vi "SequenceIndexGet.vi"(8 "error in (no error)":errorcluster, 10 "SequenceIndexName":string, 11 "VariableManager in":refnum<class "VariableManager.lvclass">) -> (0 "error out":errorcluster, 2 "SequenceIndex":refnum<class "SequenceIndex.lvclass">, 3 "VariableManager out":refnum<class "VariableManager.lvclass">)   [LabVIEW 2013, in "VariableManager.lvclass"]
doc: "Return sequence index definition of SequenceIndexName\n\nAn error is thrown if a SequenceIndexName does not exist."
uses:
  VariableManager.lvclass
  SequenceIndex/SequenceIndex.lvclass
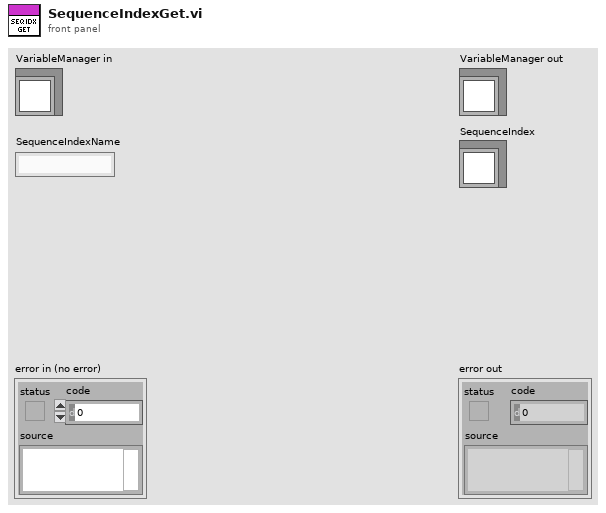
[diagram p1: front panel]
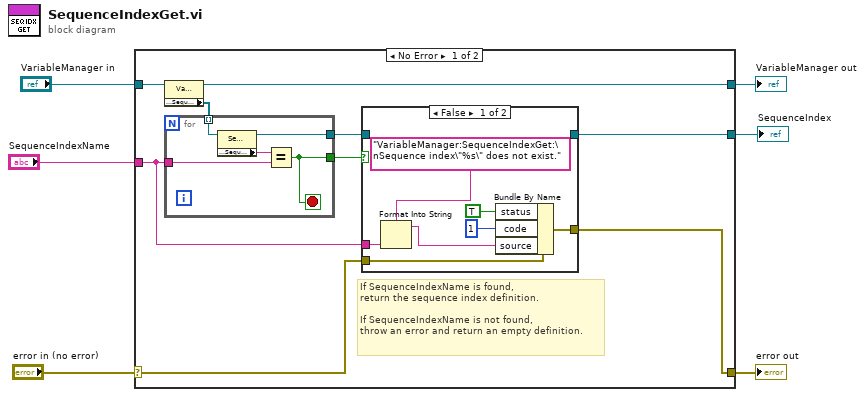
[diagram p0: block diagram]
diagram:
  n1 = case shown="No Error" "error in (no error)" {
    selector: "error in (no error)" -> [w9 w31]
    tunnel: [w7 w31] -> w5
    tunnel: [w14 w30] -> w3
    tunnel: "VariableManager in" -> [w15 w30]
    tunnel: "SequenceIndexName" -> [w8 _]
    tunnel: [w10 _] -> w1
    frame No Error {
      # "If SequenceIndexName is found, \nreturn the sequence index definition.\n\nIf SequenceIndexName is not found,\nthrow an error and return an empty definition."
      n2 = property class="VariableManager.lvclass"(reference=w15) -> (reference out=w14:refnum<class "VariableManager.lvclass">, "Accessors:SequenceIndices"=w11:refnum<class "SequenceIndex.lvclass">[])  [unwired: 1 in, 1 out]
      n3 = for {
        tunnel: w11 -> [w29] mode=indexing
        tunnel: w8 -> [w27]
        tunnel: [w26] -> w13
        tunnel: [w25] -> w12
        stop <- w26 stop-if-true
        n4 = property class="SequenceIndex.lvclass"(reference=w29) -> (reference out=w25:refnum<class "SequenceIndex.lvclass">, "Accessors:SequenceIndexName"=w28:string)  [unwired: 1 in, 1 out]
        n5 = Equal?(x=w28, y=w27) -> (x = y?=w26:bool)
      }
      n6 = case shown="False" w13 {
        tunnel: w12 -> [_ w24]
        tunnel: [_ w24] -> w10
        tunnel: w9 -> [w22 w23]
        tunnel: w8 -> [w18 _]
        tunnel: [w16 w23] -> w7
        frame False {
          n7 = Format Into String(format string="VariableManager:SequenceIndexGet:\nSequence index\"%s\" does not exist.", w18) -> (resulting string=w17:string)  [unwired: 2 in, 1 out]
          n8 = Bundle By Name(cluster=w22, "status"=TRUE, "code"=1, "source"=w17) -> (w16:errorcluster)
        }
        frame True {
        }
      }
    }
    frame Error {
    }
  }
  "error out" <- w5
  "VariableManager out" <- w3
  "SequenceIndex" <- w1
